vi "KDC101_Home.vi"(8 "error in (no error)":errorcluster caption="entrée d'erreur (pas d'erreur)", 9 "MovingRef":refnum<vi>, 10 "StopRef":refnum<vi>, 11 "KCubeDCServoRef":refnum<k24>) -> (0 "error out":errorcluster caption="sortie d'erreur", 1 "Homed":bool, 2 "ActPos(Deg)":dbl=60.0 caption="ActPos(deg)" min=0.1 step=0.1 format="%#.1f", 3 "KCubeDCServoRefOut":refnum<k24>)   [LabVIEW 2019]
doc: "Utilisez ce modèle pour construire un VI à utiliser en tant que sous-VI."
uses:
  C:/Program Files (x86)/National Instruments/LabVIEW 2019/user.lib/ThorKDC101/Kinesis_with_LabVIEW_Examples_LV12 - v3/ThorLabs.MotionControl.KCube.DCServoCLI.dll
  Kinesis_with_LabVIEW_Examples_LV12 - v3/ThorLabs.MotionControl.KCube.DCServoCLI.dll
  C:/Program Files (x86)/National Instruments/LabVIEW 2019/user.lib/ThorKDC101/Kinesis_with_LabVIEW_Examples_LV12 - v3/Thorlabs.MotionControl.GenericMotorCLI.dll
  Kinesis_with_LabVIEW_Examples_LV12 - v3/Thorlabs.MotionControl.GenericMotorCLI.dll
panel:
  in  "Stop":bool
  out "Moving":bool
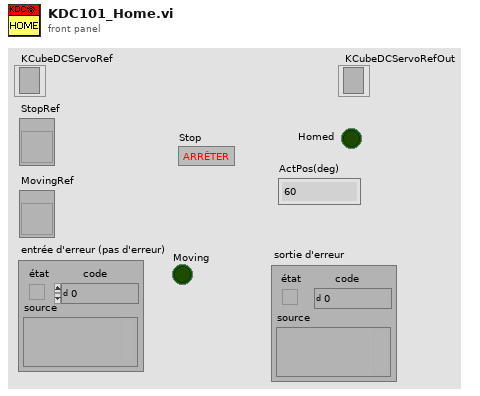
[diagram p1: front panel]
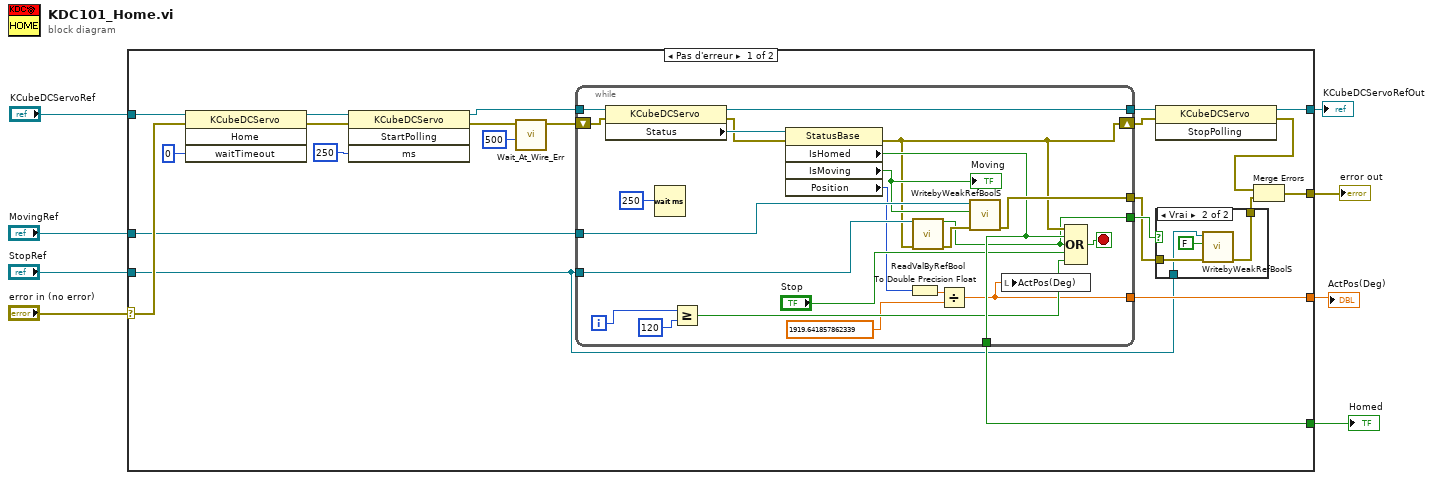
[diagram p0: block diagram]
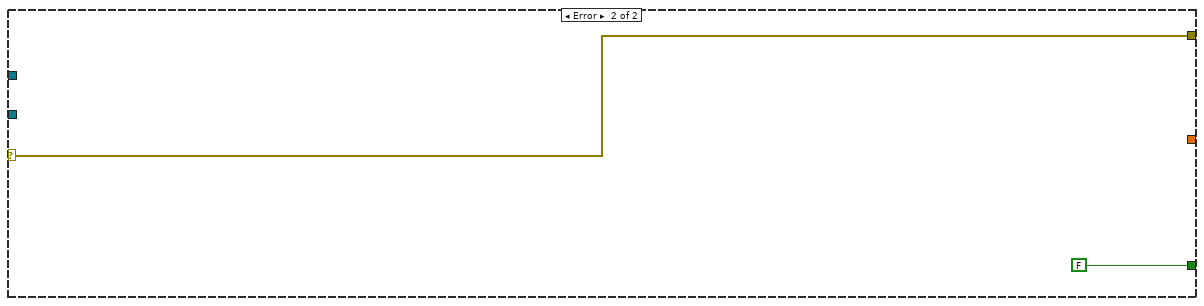
[diagram p3: hidden frame]
diagram:
  n1 = case shown="Pas d'erreur" "error in (no error)" {
    selector: "error in (no error)" -> [w25 w60]
    tunnel: [w19 w60] -> w7
    tunnel: [w18 FALSE] -> w6
    tunnel: "KCubeDCServoRef" -> [w28 _]
    tunnel: "MovingRef" -> [w20 _]
    tunnel: [w15 _] -> w3
    tunnel: "StopRef" -> [w9 _]
    tunnel: [w13 _] -> w1
    frame No Error {
      n2 = invoke class="KCubeDCServo" method="Home"(reference=w28, error in=w25, "waitTimeout"=0) -> (reference out=w23:refnum<k24>, error out=w24:errorcluster)  [unwired: 1 in, 2 out]
      n3 = invoke class="KCubeDCServo" method="StartPolling"(reference=w23, error in=w24, "ms"=250) -> (reference out=w21:refnum<k24>, error out=w22:errorcluster)  [unwired: 1 in, 2 out]
      n4 = call <userlib>:"Wait_At_Wire_Err.vi"("Wait (ms)"=u32 500, "error in (no error)"=w22) -> ("error out"=w27:errorcluster)  [unwired: 7 in, 2 out]
      n5 = while {
        tunnel: [w56] -> w16
        tunnel: w21 -> [w57]
        tunnel: w20 -> [w51]
        shift-right: [w45] -> w17
        shift-left: w27 -> [w55]
        tunnel: [w49] -> w11
        tunnel: [w48] -> w18
        tunnel: w9 -> [w47]
        tunnel: [w37] -> w13
        tunnel: [w36] -> w12
        i -> [w42]
        stop <- w52 stop-if-true
        n6 = property class="KCubeDCServo"(reference=w57, error in=w55) -> (reference out=w56:refnum<k24>, error out=w54:errorcluster, "Status"=w58:refnum<k24>)
        n7 = Wait (ms)(milliseconds to wait=u32 250) -> ()  [unwired: 1 out]
        n8 = Greater Or Equal?(x=w42, y=120 ("x")) -> (x >= y?=w44:bool)
        n9 = property class="StatusBase"(reference=w58, error in=w54) -> (error out=w45:errorcluster, "IsHomed"=w48:bool, "IsMoving"=w50:bool, "Position"=w39:i64)  [unwired: 1 out]
        "Moving" <- w50
        n10 = To Double Precision Float(number=w39) -> (double precision float=w40:dbl)
        n11 = call <userlib>:"ReadValByRefBool.vi"("Control Ref"=w47, "error in"=w45) -> ("Valeur"=w36:bool, "error out"=w46:errorcluster)  [unwired: 12 in]
        n12 = Divide(x=w40, y=1919.641857862339) -> (x/y=w37:dbl)
        n13 = call <userlib>:"WritebyWeakRefBoolS.vi"("error in"=w46, "Valeur"=w50, "Control Ref"=w51) -> ("error out"=w49:errorcluster)  [unwired: 8 in]
        n14 = local write "ActPos(Deg)"(w37) -> ()
        n15 = Compound Arithmetic op=OR ("Opérateur arithmétique")(w45, w48, w36, "Stop", w44) -> (w52:bool)
      }
      n16 = invoke class="KCubeDCServo" method="StopPolling"(reference=w16, error in=w17) -> (reference out=w15:refnum<k24>, error out=w14:errorcluster)  [unwired: 1 in, 1 out]
      n17 = case shown="Vrai" w12 {
        tunnel: w11 -> [w31 w35]
        tunnel: [w31 w34] -> w10
        tunnel: w9 -> [_ w32]
        frame False {
        }
        frame True {
          n18 = call <userlib>:"WritebyWeakRefBoolS.vi"("error in"=w35, "Valeur"=FALSE, "Control Ref"=w32) -> ("error out"=w34:errorcluster)  [unwired: 8 in]
        }
      }
      n19 = Merge Errors(w14, w10) -> (w19:errorcluster)
    }
    frame Error {
    }
  }
  "error out" <- w7
  "Homed" <- w6
  "KCubeDCServoRefOut" <- w3
  "ActPos(Deg)" <- w1
